vi "RegisterForFrameCompleteEvent_DEPRECATED.vi"(8 "error in (no error)":errorcluster, 11 "reference in":refnum<class "Camera_IMAQdx.lvclass">) -> (0 "error out":errorcluster, 2 "Frame Complete Event":refnum<event-registration>, 3 "reference in":refnum<class "Camera_IMAQdx.lvclass">)   [LabVIEW 2017]
doc: "Registers for the Frame Complete Event on an acquisition that has been started. This event will be unregistered when the acquisition is stopped automatically."
uses:
  Camera_IMAQdx.lvclass
  <vilib>/userdefined/High Color/IMAQdx.ctl
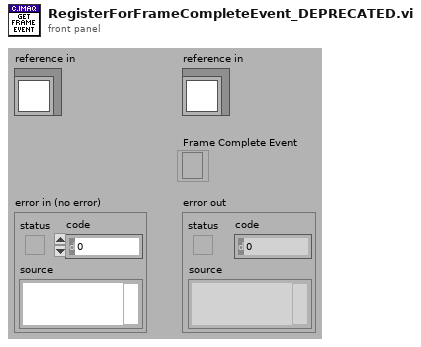
[diagram p1: front panel]
types:
  T1 = typedef "IMAQdx.ctl" = refnum<k21>
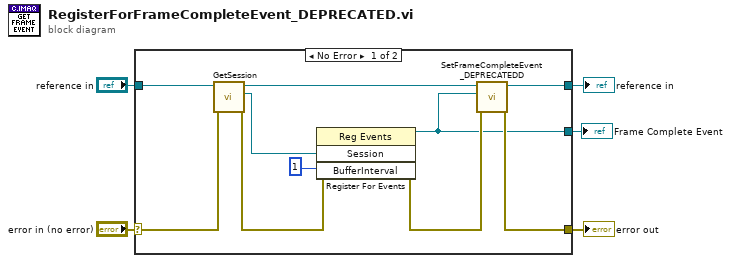
[diagram p0: block diagram]
diagram:
  n1 = case shown="No Error" "error in (no error)" {
    selector: "error in (no error)" -> [w11 w17]
    tunnel: [w7 w17] -> w4
    tunnel: [w9 w16] -> w2
    tunnel: "reference in" -> [w15 w16]
    tunnel: [w6 _] -> w1
    frame No Error {
      n2 = call "GetSession.vi"("error in (no error)"=w11, "reference in"=w15) -> ("error out"=w10:errorcluster, "Session"=w12:T1, "reference out"=w14:refnum<class "Camera_IMAQdx.lvclass">)  [unwired: 7 in]
      n3 = register-events(error in=w10, w12, u32 1 ("BufferInterval")) -> (reference out=w6:refnum<event-registration>, error out=w8:errorcluster)  [unwired: 1 in]
      n4 = call-dynamic "SetFrameCompleteEvent_DEPRECATEDD.vi"("error in (no error)"=w8, "Frame Complete Event"=w6, "reference in"=w14) -> ("error out"=w7:errorcluster, "reference in"=w9:refnum<class "Camera_IMAQdx.lvclass">)  [unwired: 7 in]
    }
    frame Error {
    }
  }
  "error out" <- w4
  "reference in" <- w2
  "Frame Complete Event" <- w1
